vi "DO_所有参数读取.vi"(5 "大气压补偿":dbl, 7 "盐度补偿":dbl, 8 "error in (no error)":errorcluster caption="错误输入（无错误）", 11 "MB session in":refnum<class "MB_Master.lvclass">) -> (0 "error out":errorcluster caption="错误输出", 2 "输出值":T1 {"电极型号标志" items=["NULL", "pH", "Cond", "DO", "Turb"]; "电极状态标志" items=["OK"]}, 3 "MB session out":refnum<class "MB_Master.lvclass">)   [LabVIEW 2016, in "斯坦道多参数.lvlib"]
uses:
  <vilib>/Plasmionique/MB Master/MB_Master/MB_Master.lvclass
  <vilib>/Plasmionique/MB Master/MB Master.lvlib
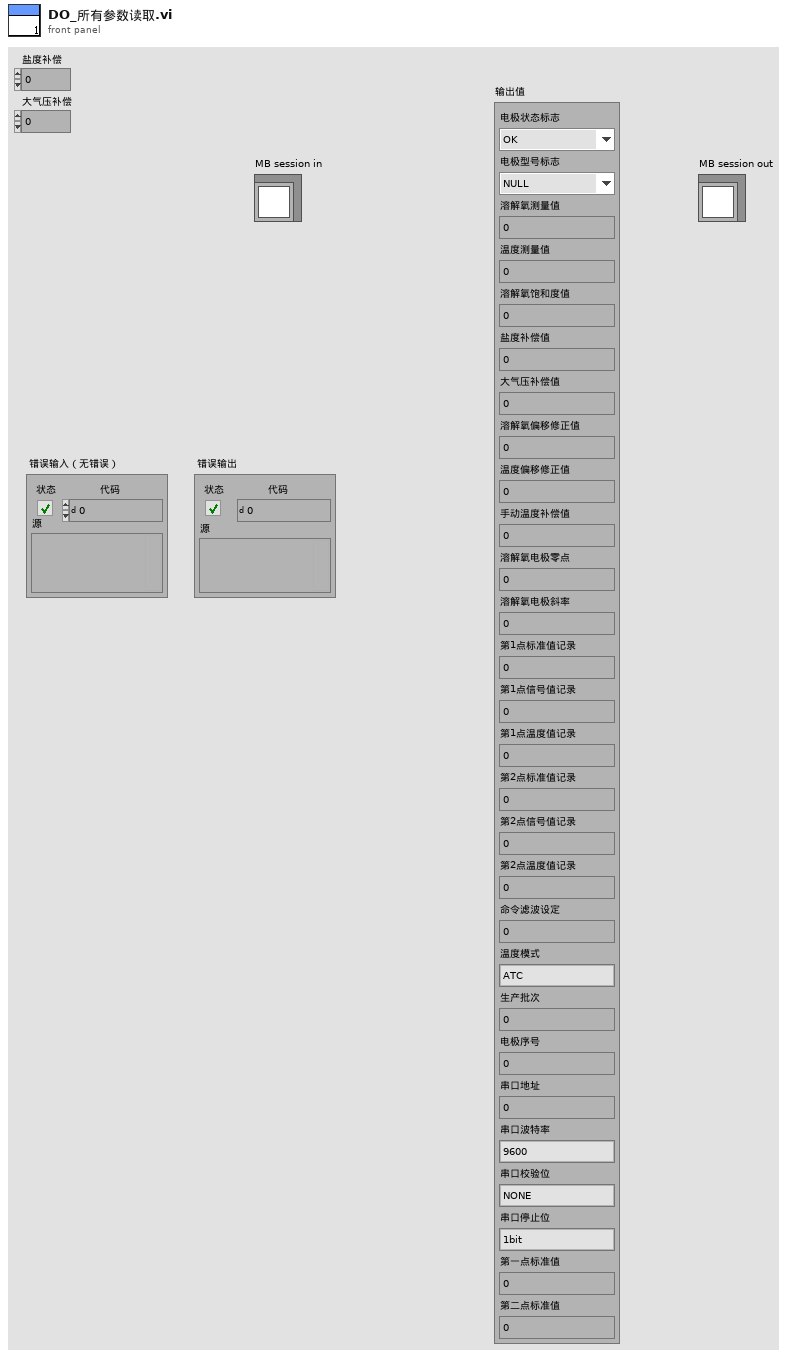
[diagram p1: front panel]
types:
  T1 = cluster{"电极状态标志":u16, "电极型号标志":u16, "溶解氧测量值":sgl, "温度测量值":sgl, "溶解氧饱和度值":sgl, "盐度补偿值":sgl, "大气压补偿值":sgl, "溶解氧偏移修正值":sgl, "温度偏移修正值":sgl, "手动温度补偿值":sgl, "溶解氧电极零点":sgl, "溶解氧电极斜率":sgl, "第1点标准值记录":sgl, "第1点信号值记录":sgl, "第1点温度值记录":sgl, "第2点标准值记录":sgl, "第2点信号值记录":sgl, "第2点温度值记录":sgl, "命令滤波设定":u16, "温度模式":enum16{"ATC", "MTC"}, "生产批次":u16, "电极序号":u16, "串口地址":u16, "串口波特率":enum16{"9600", "19200", "115200"}, "串口校验位":enum16{"NONE", "ODD", "EVEN"}, "串口停止位":enum16{"1bit", "2bit"}, "第一点标准值":sgl, "第二点标准值":sgl}
  T2 = cluster{u16, u16, "DataDo_mgL":dbl, "数值":sgl, "数值":sgl, "盐度补偿":dbl, "大气压补偿":dbl, "数值":sgl, "数值":sgl, "数值":sgl, "数值":sgl, "数值":sgl, "数值":sgl, "数值":sgl, "数值":sgl, "数值":sgl, "数值":sgl, "数值":sgl, u16, u16, u16, u16, u16, u16, u16, u16, "数值":sgl, "数值":sgl}
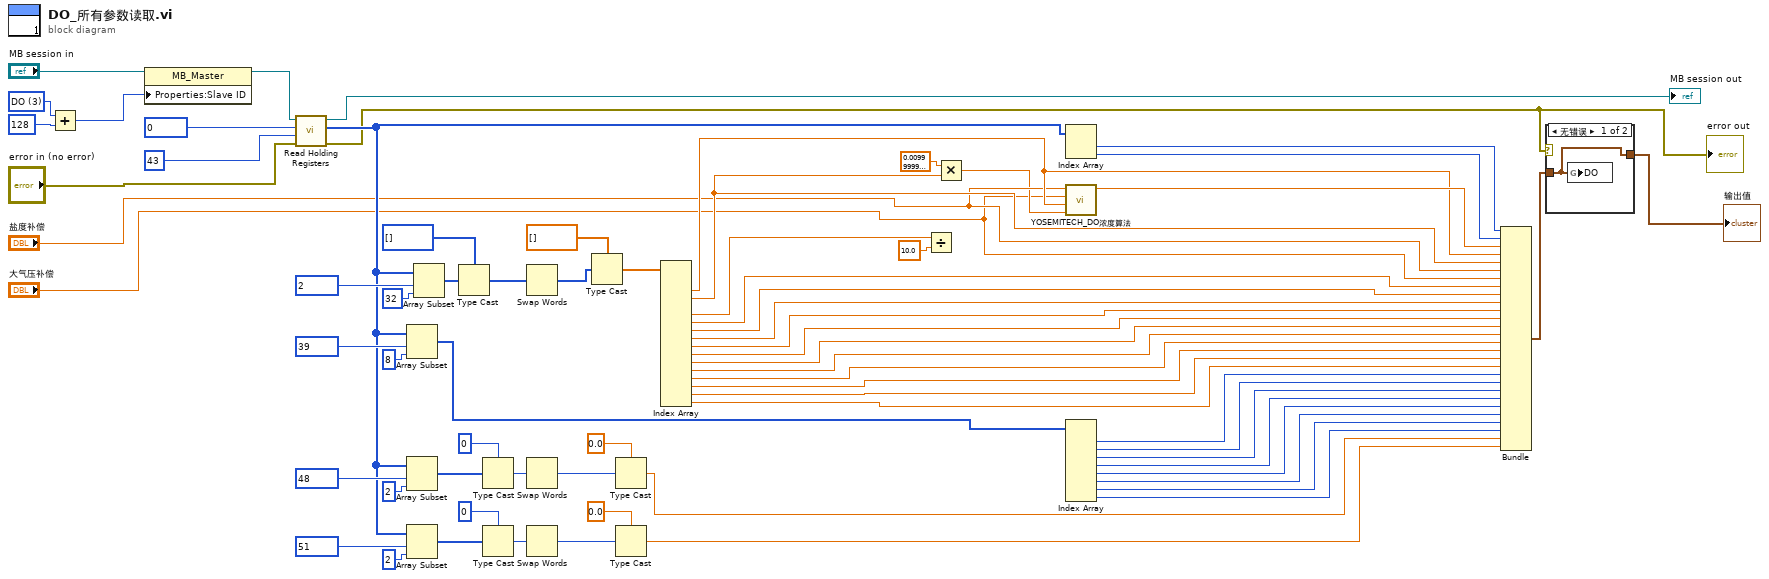
[diagram p0: block diagram]
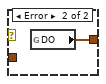
[diagram p2: hidden frame]
diagram:
  w70 = u16 3 items=["NULL", "pH", "Cond", "DO", "Turb"] ("数值")
  n1 = Add(x=w70, y=u16 128) -> (x+y=w69:u16)
  n2 = property class="MB_Master"(reference="MB session in", "Properties:Slave ID"=w69) -> (reference out=w15:refnum<class "MB_Master.lvclass">)  [unwired: 1 in, 1 out]
  n3 = call <vilib>:"Read Holding Registers.vi"("error in (no error)"="error in (no error)", "quantity"=u16 43, "starting address"=u16 0, "MB session in"=w15) -> ("error out"=w14:errorcluster, "Registers"=w29:u16[], "MB session out"=→"MB session out":refnum<class "MB_Master.lvclass">)  [unwired: 5 in]
  "error out" <- w14
  n4 = Array Subset(array=w29, index=u16 39 ("starting address"), length=8 ("长度")) -> (w42:u16[])
  n5 = Array Subset(array=w29, index=u16 48 ("starting address"), length=2 ("长度")) -> (w24:u16[])
  n6 = Array Subset(array=w29, index=u16 51 ("starting address"), length=2 ("长度")) -> (w19:u16[])
  n7 = Array Subset(array=w29, index=u16 2 ("starting address"), length=32 ("长度")) -> (w58:u16[])
  n8 = Type Cast(type=u32[] [] ("数组 2"), x=w58) -> (*(type *) &x=w61:u32[])
  n9 = Type Cast(type=u32 0 ("数值"), x=w24) -> (*(type *) &x=w27:u32)
  n10 = Type Cast(type=u32 0 ("数值"), x=w19) -> (*(type *) &x=w21:u32)
  n11 = Swap Words(1:w61) -> (0:w62:u32[])
  n12 = Swap Words(1:w27) -> (0:w28:u32)
  n13 = Swap Words(1:w21) -> (0:w20:u32)
  n14 = Type Cast(type=sgl[] [] ("数组 2"), x=w62) -> (*(type *) &x=w57:sgl[])
  n15 = Type Cast(type=sgl 0.0 ("数值"), x=w28) -> (*(type *) &x=w18:sgl)
  n16 = Type Cast(type=sgl 0.0 ("数值"), x=w20) -> (*(type *) &x=w17:sgl)
  n17 = Index Array(array=w57) -> (element #2=w9:sgl, element #3=w8:sgl, element #5=w6:sgl, element #6=w56:sgl, element #7=w55:sgl, element #8=w54:sgl, element #9=w53:sgl, element #10=w52:sgl, element #11=w51:sgl, element #12=w50:sgl, element #13=w49:sgl, element #14=w48:sgl, element #15=w47:sgl, element #16=w46:sgl)  [unwired: 16 in, 2 out]
  n18 = Divide(x=w6, y=sgl 10.0) -> ()  [unwired: 1 out]
  n19 = Multiply(x=sgl 0.01, y=w8) -> (x*y=w4:sgl)
  n20 = Index Array(array=w29) -> (element #1=w65:u16, element #2=w64:u16)  [unwired: 2 in]
  n21 = call "YOSEMITECH_DO浓度算法.vi"("溶解氧饱和度值"=w4, "水温"=w9, "大气压补偿"="大气压补偿", "盐度补偿"="盐度补偿") -> ("DataDo_mgL"=w10:dbl)  [unwired: 7 in]
  n22 = Index Array(array=w42) -> (element #1=w41:u16, element #2=w40:u16, element #3=w39:u16, element #4=w38:u16, element #5=w37:u16, element #6=w36:u16, element #7=w35:u16, element #8=w34:u16)  [unwired: 8 in]
  n23 = Bundle(w65, w64, "DataDo_mgL"=w10, "数值"=w9, "数值"=w8, "盐度补偿"="盐度补偿", "大气压补偿"="大气压补偿", "数值"=w56, "数值"=w55, "数值"=w54, "数值"=w53, "数值"=w52, "数值"=w51, "数值"=w50, "数值"=w49, "数值"=w48, "数值"=w47, "数值"=w46, w41, w40, w39, w38, w37, w36, w35, w34, "数值"=w18, "数值"=w17) -> (w13:T2)  [unwired: 1 in]
  n24 = case shown="无错误" w14 {
    tunnel: w13 -> [w71 _]
    tunnel: [w71 w72] -> w2
    frame No Error {
      n25 = global write "国弘过程全局变量.vi" "DO"(w71) -> ()
    }
    frame Error {
      n26 = global read "国弘过程全局变量.vi" "DO"() -> (w72:T1)
    }
  }
  "输出值" <- w2
